vi "Equi-Ripple HighPass.vi"   [LabVIEW 2020, in "NI_AALBase.lvlib"]
doc: "Generates a highpass FIR filter with equi-ripple characteristics using the Parks-McClellan algorithm and the <B># of taps</B>, <B>stop freq</B>, <B>high freq</B>, and <B>sampling freq: fs</B>. The Equi-Ripple HighPass VI then applies a linear-phase, highpass filter to the input sequence <B>X</B> using the Convolution VI to obtain <B>Filtered X</B>. Wire data to the <B>X</B> input to determine the polymorphic instance to use or manually select the instance."
uses:
  <vilib>/Analysis/NI_AALBase.lvlib
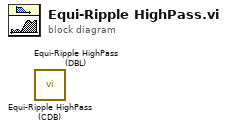
[diagram p0: block diagram]
diagram:
  n1 = call <vilib>:"Equi-Ripple HighPass (CDB).vi"() -> ()  [unwired: 6 in, 2 out]
  n2 = call <vilib>:"Equi-Ripple HighPass (DBL).vi"() -> ()  [unwired: 6 in, 2 out]
